vi "Open Project.vi"(6 "Open Window?":bool, 8 "error in (no error)":errorcluster, 11 "Build Project":path) -> (0 "error out":errorcluster, 3 "Project out":refnum<vi>)   [LabVIEW 2018]
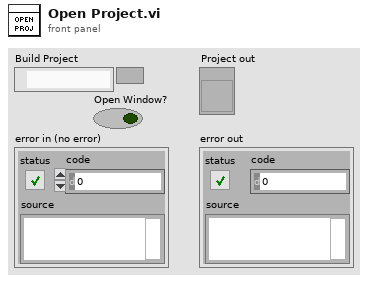
[diagram p1: front panel]
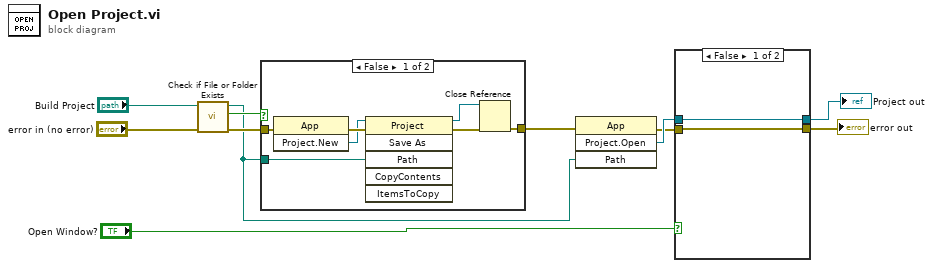
[diagram p0: block diagram]
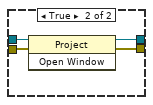
[diagram p2: hidden frame]
diagram:
  n1 = call <vilib>:"Check if File or Folder Exists.vi"("error in (no error)"="error in (no error)", "path"="Build Project") -> ("error out"=w8:errorcluster, "file or folder exists?"=w9:bool, "dup path"=w7:path)  [unwired: 7 in]
  n2 = case shown="False" w9 {
    tunnel: [w14 w19] -> w6
    tunnel: w7 -> [w13 _]
    tunnel: w8 -> [w12 w19]
    frame False {
      n3 = invoke class="App" method="Project.New"(error in=w12) -> (error out=w18:errorcluster, "Project:New"=w17:refnum<vi>)  [unwired: 2 in, 1 out]
      n4 = invoke class="Project" method="Save As"(reference=w17, error in=w18, "Path"=w13) -> (reference out=w15:refnum<vi>, error out=w16:errorcluster)  [unwired: 3 in, 4 out]
      n5 = Close Reference(reference=w15, error in (no error)=w16) -> (error out=w14:errorcluster)
    }
    frame True {
    }
  }
  n6 = invoke class="App" method="Project.Open"(error in=w6, "Path"=w7) -> (error out=w3:errorcluster, "Project:Open"=w5:refnum<vi>)  [unwired: 2 in, 2 out]
  n7 = case shown="False" "Open Window?" {
    tunnel: w5 -> [w21 w25]
    tunnel: [w21 w24] -> w4
    tunnel: w3 -> [w20 w23]
    tunnel: [w20 w22] -> w2
    frame False {
    }
    frame True {
      n8 = invoke class="Project" method="Open Window"(reference=w25, error in=w23) -> (reference out=w24:refnum<vi>, error out=w22:errorcluster)  [unwired: 1 in, 1 out]
    }
  }
  "Project out" <- w4
  "error out" <- w2
